vi "Write Client type.vi"(8 "error in (no error)":errorcluster, 10 "Client type":enum16{"Control", "Reciever", "Transmitter"}(ring), 11 "RP Instrument in":refnum<class "RP Instrument.lvclass">) -> (0 "error out":errorcluster, 3 "RP Instrument out":refnum<class "RP Instrument.lvclass">)   [LabVIEW 2015, in "RP Instrument.lvclass"]
uses:
  RP Instrument.lvclass
  RP Instrument.lvclass/RP Instrument.ctl
  RP Communicator/RP Communicator.lvclass/RP Communicator.ctl
  RP Communicator/RP Communicator.lvclass
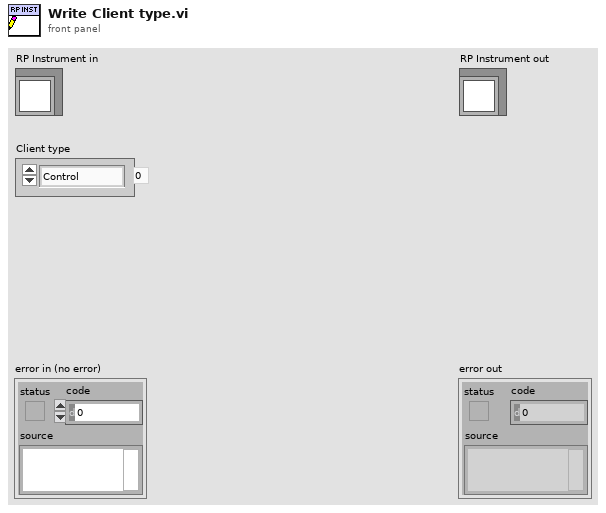
[diagram p1: front panel]
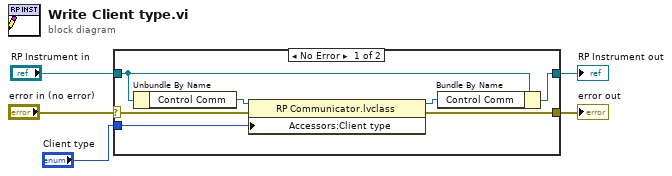
[diagram p0: block diagram]
diagram:
  n1 = case shown="No Error" "error in (no error)" {
    selector: "error in (no error)" -> [w7 w13]
    tunnel: [w6 w13] -> w4
    tunnel: [w12 w14] -> w2
    tunnel: "RP Instrument in" -> [w11 w14]
    tunnel: "Client type" -> [w8 _]
    frame No Error {
      n2 = Unbundle By Name(w11) -> ("Control Comm"=w10:refnum<class "RP Communicator.lvclass">)
      n3 = property class="RP Communicator.lvclass"(reference=w10, error in=w7, "Accessors:Client type"=w8) -> (reference out=w9:refnum<class "RP Communicator.lvclass">, error out=w6:errorcluster)
      n4 = Bundle By Name(cluster=w11, "Control Comm"=w9) -> (w12:refnum<class "RP Instrument.lvclass">)
    }
    frame Error {
    }
  }
  "error out" <- w4
  "RP Instrument out" <- w2
